vi "getInstrAbbr.vi"(1 "ctlarr":T1) -> (0 "abbrArray":string[](array[string]))   [LabVIEW 2017]
uses:
  RefArray/RefArray.ctl
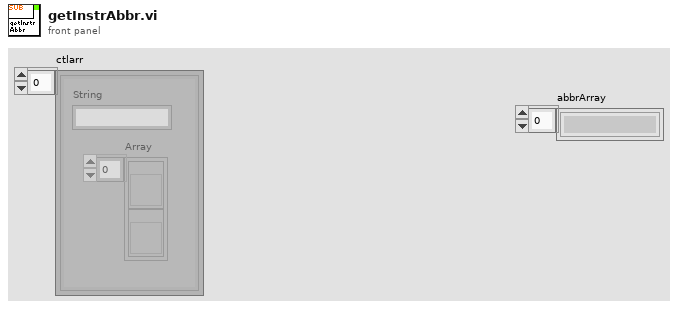
[diagram p1: front panel]
types:
  T1 = typedef "RefArray.ctl" = cluster{"String":string, "Array":refnum<vi>[]}[]
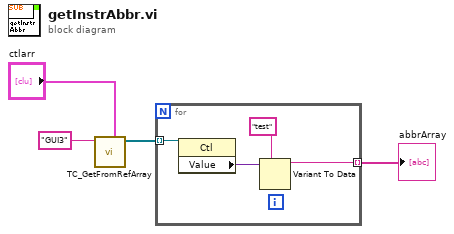
[diagram p0: block diagram]
diagram:
  n1 = call "TC_GetFromRefArray.vi"("arrayIn"="ctlarr", "NameToFind"="GUI3") -> ("refArray"=w2:refnum<vi>[])  [unwired: 8 in, 1 out]
  n2 = for {
    tunnel: w2 -> [w8] mode=indexing
    tunnel: [w6] -> w1 mode=indexing
    n3 = property class="Ctl"(reference=w8) -> ("Value"=w7:variant)  [unwired: 1 in, 2 out]
    n4 = Variant To Data(type="test", Variant=w7) -> (data=w6:string)  [unwired: 1 in, 1 out]
  }
  "abbrArray" <- w1
